vi "example_02_convert.vi"() -> ()   [LabVIEW 2015, in "lv-unit-conversion.lvlib"] (continued)
"d"=0.0, "underlying_def"="", "description"=""}, {"symbol"="GS", "name"="gigasiemens", "dimension"="I2T3/L2M", "is_si_unit"=TRUE, "category"="prefixed", "base_unit"="S", "conversion_reference"="DERIVED", "is_exact"=TRUE, "a"=0.0, "b"=1000000000.0, "c"=1.0, "d"=0.0, "underlying_def"="", "description"=""}, {"symbol"="kS", "name"="kilosiemens", "dimension"="I2T3/L2M", "is_si_unit"=TRUE, "category"="prefixed", "base_unit"="S", "conversion_reference"="DERIVED", "is_exact"=TRUE, "a"=0.0, "b"=1000.0, "c"=1.0, "d"=0.0, "underlying_def"="", "description"=""}, {"symbol"="mS", "name"="millisiemens", "dimension"="I2T3/L2M", "is_si_unit"=TRUE, "category"="prefixed", "base_unit"="S", "conversion_reference"="DERIVED", "is_exact"=TRUE, "a"=0.0, "b"=0.001, "c"=1.0, "d"=0.0, "underlying_def"="", "description"=""}, {"symbol"="MS", "name"="megasiemens", "dimension"="I2T3/L2M", "is_si_unit"=TRUE, "category"="prefixed", "base_unit"="S", "conversion_reference"="DERIVED", "is_exact"=TRUE, "a"=0.0, "b"=1000000.0, "c"=1.0, "d"=0.0, "underlying_def"="", "description"=""}, {"symbol"="nS", "name"="nanosiemens", "dimension"="I2T3/L2M", "is_si_unit"=TRUE, "category"="prefixed", "base_unit"="S", "conversion_reference"="DERIVED", "is_exact"=TRUE, "a"=0.0, "b"=1e-09, "c"=1.0, "d"=0.0, "underlying_def"="", "description"=""}, {"symbol"="pS", "name"="picosiemens", "dimension"="I2T3/L2M", "is_si_unit"=TRUE, "category"="prefixed", "base_unit"="S", "conversion_reference"="DERIVED", "is_exact"=TRUE, "a"=0.0, "b"=1e-12, "c"=1.0, "d"=0.0, "underlying_def"="", "description"=""}, {"symbol"="TS", "name"="terasiemens", "dimension"="I2T3/L2M", "is_si_unit"=TRUE, "category"="prefixed", "base_unit"="S", "conversion_reference"="DERIVED", "is_exact"=TRUE, "a"=0.0, "b"=1000000000000.0, "c"=1.0, "d"=0.0, "underlying_def"="", "description"=""}, {"symbol"="uS", "name"="microsiemens", "dimension"="I2T3/L2M", "is_si_unit"=TRUE, "category"="prefixed", "base_unit"="S", "conversion_reference"="DERIVED", "is_exact"=TRUE, "a"=0.0, "b"=1e-06, "c"=1.0, "d"=0.0, "underlying_def"="", "description"=""}, {"symbol"="S/m", "name"="siemens per metre", "dimension"="I2T3/L3M", "is_si_unit"=TRUE, "category"="derived", "base_unit"="", "conversion_reference"="", "is_exact"=FALSE, "a"=0.0, "b"=0.0, "c"=0.0, "d"=0.0, "underlying_def"="", "description"=""}, {"symbol"="kS/m", "name"="kilosiemens per metre", "dimension"="I2T3/L3M", "is_si_unit"=TRUE, "category"="derived", "base_unit"="S/m", "conversion_reference"="DERIVED", "is_exact"=TRUE, "a"=0.0, "b"=1000.0, "c"=1.0, "d"=0.0, "underlying_def"="", "description"=""}, {"symbol"="mS/cm", "name"="millisiemens per centimetre", "dimension"="I2T3/L3M", "is_si_unit"=TRUE, "category"="derived", "base_unit"="S/m", "conversion_reference"="DERIVED", "is_exact"=TRUE, "a"=0.0, "b"=0.1, "c"=1.0, "d"=0.0, "underlying_def"="", "description"=""}, {"symbol"="mS/m", "name"="millisiemens per metre", "dimension"="I2T3/L3M", "is_si_unit"=TRUE, "category"="derived", "base_unit"="S/m", "conversion_reference"="DERIVED", "is_exact"=TRUE, "a"=0.0, "b"=0.001, "c"=1.0, "d"=0.0, "underlying_def"="", "description"=""}, {"symbol"="F", "name"="farad", "dimension"="I2T4/L2M", "is_si_unit"=TRUE, "category"="atom-special", "base_unit"="", "conversion_reference"="", "is_exact"=FALSE, "a"=0.0, "b"=0.0, "c"=0.0, "d"=0.0, "underlying_def"="C/V", "description"="The capacitance of a capacitor between the plates of which there appears a difference of potential \n\t\t\t\tof 1 V when it is charged by a quantity of electricity equal to 1 C.\n\t\t\t"}, {"symbol"="cF", "name"="centifarad", "dimension"="I2T4/L2M", "is_si_unit"=TRUE, "category"="prefixed", "base_unit"="F", "conversion_reference"="DERIVED", "is_exact"=TRUE, "a"=0.0, "b"=0.01, "c"=1.0, "d"=0.0, "underlying_def"="", "description"=""}, {"symbol"="dF", "name"="decifarad", "dimension"="I2T4/L2M", "is_si_unit"=TRUE, "category"="prefixed", "base_unit"="F", "conversion_reference"="DERIVED", "is_exact"=TRUE, "a"=0.0, "b"=0.1, "c"=1.0, "d"=0.0, "underlying_def"="", "description"=""}, {"symbol"="EF", "name"="exafarad", "dimension"="I2T4/L2M", "is_si_unit"=TRUE, "category"="prefixed", "base_unit"="F", "conversion_reference"="DERIVED", "is_exact"=TRUE, "a"=0.0, "b"=1e+18, "c"=1.0, "d"=0.0, "underlying_def"="", "description"=""}, {"symbol"="fF", "name"="femtofarad", "dimension"="I2T4/L2M", "is_si_unit"=TRUE, "category"="prefixed", "base_unit"="F", "conversion_reference"="DERIVED", "is_exact"=TRUE, "a"=0.0, "b"=1e-15, "c"=1.0, "d"=0.0, "underlying_def"="", "description"=""}, {"symbol"="GF", "name"="gigafarad", "dimension"="I2T4/L2M", "is_si_unit"=TRUE, "category"="prefixed", "base_unit"="F", "conversion_reference"="DERIVED", "is_exact"=TRUE, "a"=0.0, "b"=1000000000.0, "c"=1.0, "d"=0.0, "underlying_def"="", "description"=""}, {"symbol"="kF", "name"="kilofarad", "dimension"="I2T4/L2M", "is_si_unit"=TRUE, "category"="prefixed", "base_unit"="F", "conversion_reference"="DERIVED", "is_exact"=TRUE, "a"=0.0, "b"=1000.0, "c"=1.0, "d"=0.0, "underlying_def"="", "description"=""}, {"symbol"="mF", "name"="millifarad", "dimension"="I2T4/L2M", "is_si_unit"=TRUE, "category"="prefixed", "base_unit"="F", "conversion_reference"="DERIVED", "is_exact"=TRUE, "a"=0.0, "b"=0.001, "c"=1.0, "d"=0.0, "underlying_def"="", "description"=""}, {"symbol"="MF", "name"="megafarad", "dimension"="I2T4/L2M", "is_si_unit"=TRUE, "category"="prefixed", "base_unit"="F", "conversion_reference"="DERIVED", "is_exact"=TRUE, "a"=0.0, "b"=1000000.0, "c"=1.0, "d"=0.0, "underlying_def"="", "description"=""}, {"symbol"="nF", "name"="nanofarad", "dimension"="I2T4/L2M", "is_si_unit"=TRUE, "category"="prefixed", "base_unit"="F", "conversion_reference"="DERIVED", "is_exact"=TRUE, "a"=0.0, "b"=1e-09, "c"=1.0, "d"=0.0, "underlying_def"="", "description"=""}, {"symbol"="pF", "name"="picofarad", "dimension"="I2T4/L2M", "is_si_unit"=TRUE, "category"="prefixed", "base_unit"="F", "conversion_reference"="DERIVED", "is_exact"=TRUE, "a"=0.0, "b"=1e-12, "c"=1.0, "d"=0.0, "underlying_def"="", "description"=""}, {"symbol"="TF", "name"="terafarad", "dimension"="I2T4/L2M", "is_si_unit"=TRUE, "category"="prefixed", "base_unit"="F", "conversion_reference"="DERIVED", "is_exact"=TRUE, "a"=0.0, "b"=1000000000000.0, "c"=1.0, "d"=0.0, "underlying_def"="", "description"=""}, {"symbol"="uF", "name"="microfarad", "dimension"="I2T4/L2M", "is_si_unit"=TRUE, "category"="prefixed", "base_unit"="F", "conversion_reference"="DERIVED", "is_exact"=TRUE, "a"=0.0, "b"=1e-06, "c"=1.0, "d"=0.0, "underlying_def"="", "description"=""}, {"symbol"="uF/m", "name"="microfarad per metre", "dimension"="I2T4/L3M", "is_si_unit"=TRUE, "category"="derived", "base_unit"="F/m", "conversion_reference"="DERIVED", "is_exact"=TRUE, "a"=0.0, "b"=1e-06, "c"=1.0, "d"=0.0, "underlying_def"="", "description"=""}, {"symbol"="F/m", "name"="farad per metre", "dimension"="I2T4/L3M", "is_si_unit"=TRUE, "category"="derived", "base_unit"="", "conversion_reference"="", "is_exact"=FALSE, "a"=0.0, "b"=0.0, "c"=0.0, "d"=0.0, "underlying_def"="", "description"=""}, {"symbol"="A.m2", "name"="ampere square metre", "dimension"="IL2", "is_si_unit"=TRUE, "category"="derived", "base_unit"="", "conversion_reference"="", "is_exact"=FALSE, "a"=0.0, "b"=0.0, "c"=0.0, "d"=0.0, "underlying_def"="", "description"=""}, {"symbol"="C.m", "name"="coulomb metre", "dimension"="ILT", "is_si_unit"=TRUE, "category"="derived", "base_unit"="", "conversion_reference"="", "is_exact"=FALSE, "a"=0.0, "b"=0.0, "c"=0.0, "d"=0.0, "underlying_def"="", "description"=""}, {"symbol"="C", "name"="coulomb", "dimension"="IT", "is_si_unit"=TRUE, "category"="atom-special", "base_unit"="", "conversion_reference"="", "is_exact"=FALSE, "a"=0.0, "b"=0.0, "c"=0.0, "d"=0.0, "underlying_def"="A.s", "description"="The time integral of electric current, equal to 1 A.s"}, {"symbol"="A.h", "name"="ampere hour", "dimension"="IT", "is_si_unit"=TRUE, "category"="derived", "base_unit"="C", "conversion_reference"="DERIVED", "is_exact"=TRUE, "a"=0.0, "b"=3600.0, "c"=1.0, "d"=0.0, "underlying_def"="", "description"=""}, {"symbol"="A.s", "name"="ampere second", "dimension"="IT", "is_si_unit"=TRUE, "category"="derived", "base_unit"="C", "conversion_reference"="DERIVED", "is_exact"=TRUE, "a"=0.0, "b"=1.0, "c"=1.0, "d"=0.0, "underlying_def"="", "description"=""}, {"symbol"="cC", "name"="centicoulomb", "dimension"="IT", "is_si_unit"=TRUE, "category"="prefixed", "base_unit"="C", "conversion_reference"="DERIVED", "is_exact"=TRUE, "a"=0.0, "b"=0.01, "c"=1.0, "d"=0.0, "underlying_def"="", "description"=""}, {"symbol"="dC", "name"="decicoulomb", "dimension"="IT", "is_si_unit"=TRUE, "category"="prefixed", "base_unit"="C", "conversion_reference"="DERIVED", "is_exact"=TRUE, "a"=0.0, "b"=0.1, "c"=1.0, "d"=0.0, "underlying_def"="", "description"=""}, {"symbol"="EC", "name"="exacoulomb", "dimension"="IT", "is_si_unit"=TRUE, "category"="prefixed", "base_unit"="C", "conversion_reference"="DERIVED", "is_exact"=TRUE, "a"=0.0, "b"=1e+18, "c"=1.0, "d"=0.0, "underlying_def"="", "description"=""}, {"symbol"="fC", "name"="femtocoulomb", "dimension"="IT", "is_si_unit"=TRUE, "category"="prefixed", "base_unit"="C", "conversion_reference"="DERIVED", "is_exact"=TRUE, "a"=0.0, "b"=1e-15, "c"=1.0, "d"=0.0, "underlying_def"="", "description"=""}, {"symbol"="GC", "name"="gigacoulomb", "dimension"="IT", "is_si_unit"=TRUE, "category"="prefixed", "base_unit"="C", "conversion_reference"="DERIVED", "is_exact"=TRUE, "a"=0.0, "b"=1000000000.0, "c"=1.0, "d"=0.0, "underlying_def"="", "description"=""}, {"symbol"="kC", "name"="kilocoulomb", "dimension"="IT", "is_si_unit"=TRUE, "category"="prefixed", "base_unit"="C", "conversion_reference"="DERIVED", "is_exact"=TRUE, "a"=0.0, "b"=1000.0, "c"=1.0, "d"=0.0, "underlying_def"="", "description"=""}, {"symbol"="mC", "name"="millicoulomb", "dimension"="IT", "is_si_unit"=TRUE, "category"="prefixed", "base_unit"="C", "conversion_reference"="DERIVED", "is_exact"=TRUE, "a"=0.0, "b"=0.001, "c"=1.0, "d"=0.0, "underlying_def"="", "description"=""}, {"symbol"="MC", "name"="megacoulomb", "dimension"="IT", "is_si_unit"=TRUE, "category"="prefixed", "base_unit"="C", "conversion_reference"="DERIVED", "is_exact"=TRUE, "a"=0.0, "b"=1000000.0, "c"=1.0, "d"=0.0, "underlying_def"="", "description"=""}, {"symbol"="nC", "name"="nanocoulomb", "dimension"="IT", "is_si_unit"=TRUE, "category"="prefixed", "base_unit"="C", "conversion_reference"="DERIVED", "is_exact"=TRUE, "a"=0.0, "b"=1e-09, "c"=1.0, "d"=0.0, "underlying_def"="", "description"=""}, {"symbol"="pC", "name"="picocoulomb", "dimension"="IT", "is_si_unit"=TRUE, "category"="prefixed", "base_unit"="C", "conversion_reference"="DERIVED", "is_exact"=TRUE, "a"=0.0, "b"=1e-12, "c"=1.0, "d"=0.0, "underlying_def"="", "description"=""}, {"symbol"="TC", "name"="teracoulomb", "dimension"="IT", "is_si_unit"=TRUE, "category"="prefixed", "base_unit"="C", "conversion_reference"="DERIVED", "is_exact"=TRUE, "a"=0.0, "b"=1000000000000.0, "c"=1.0, "d"=0.0, "underlying_def"="", "description"=""}, {"symbol"="uC", "name"="microcoulomb", "dimension"="IT", "is_si_unit"=TRUE, "category"="prefixed", "base_unit"="C", "conversion_reference"="DERIVED", "is_exact"=TRUE, "a"=0.0, "b"=1e-06, "c"=1.0, "d"=0.0, "underlying_def"="", "description"=""}, {"symbol"="C/cm2", "name"="coulomb per square centimetre", "dimension"="IT/L2", "is_si_unit"=TRUE, "category"="derived", "base_unit"="C/m2", "conversion_reference"="DERIVED", "is_exact"=TRUE, "a"=0.0, "b"=10000.0, "c"=1.0, "d"=0.0, "underlying_def"="", "description"=""}, {"symbol"="C/mm2", "name"="coulomb per square millimetre", "dimension"="IT/L2", "is_si_unit"=TRUE, "category"="derived", "base_unit"="C/m2", "conversion_reference"="DERIVED", "is_exact"=TRUE, "a"=0.0, "b"=1000000.0, "c"=1.0, "d"=0.0, "underlying_def"="", "description"=""}, {"symbol"="mC/m2", "name"="millicoulomb per square metre", "dimension"="IT/L2", "is_si_unit"=TRUE, "category"="derived", "base_unit"="C/m2", "conversion_reference"="DERIVED", "is_exact"=TRUE, "a"=0.0, "b"=0.001, "c"=1.0, "d"=0.0, "underlying_def"="", "description"=""}, {"symbol"="C/m2", "name"="coulomb per square metre", "dimension"="IT/L2", "is_si_unit"=TRUE, "category"="derived", "base_unit"="", "conversion_reference"="", "is_exact"=FALSE, "a"=0.0, "b"=0.0, "c"=0.0, "d"=0.0, "underlying_def"="", "description"=""}, {"symbol"="A.s/m3", "name"="ampere second per cubic metre", "dimension"="IT/L3", "is_si_unit"=TRUE, "category"="derived", "base_unit"="C/m3", "conversion_reference"="DERIVED", "is_exact"=TRUE, "a"=0.0, "b"=1.0, "c"=1.0, "d"=0.0, "underlying_def"="", "description"=""}, {"symbol"="C/cm3", "name"="coulomb per cubic centimetre", "dimension"="IT/L3", "is_si_unit"=TRUE, "category"="derived", "base_unit"="C/m3", "conversion_reference"="DERIVED", "is_exact"=TRUE, "a"=0.0, "b"=1000000.0, "c"=1.0, "d"=0.0, "underlying_def"="", "description"=""}, {"symbol"="C/mm3", "name"="coulomb per cubic millimetre", "dimension"="IT/L3", "is_si_unit"=TRUE, "category"="derived", "base_unit"="C/m3", "conversion_reference"="DERIVED", "is_exact"=TRUE, "a"=0.0, "b"=1000000000.0, "c"=1.0, "d"=0.0, "underlying_def"="", "description"=""}, {"symbol"="C/m3", "name"="coulomb per cubic metre", "dimension"="IT/L3", "is_si_unit"=TRUE, "category"="derived", "base_unit"="", "conversion_reference"="", "is_exact"=FALSE, "a"=0.0, "b"=0.0, "c"=0.0, "d"=0.0, "underlying_def"="", "description"=""}, {"symbol"="A.s/kg", "name"="ampere second per kilogram", "dimension"="IT/M", "is_si_unit"=TRUE, "category"="derived", "base_unit"="C/kg", "conversion_reference"="DERIVED", "is_exact"=TRUE, "a"=0.0, "b"=1.0, "c"=1.0, "d"=0.0, "underlying_def"="", "description"=""}, {"symbol"="C/g", "name"="coulomb per gram", "dimension"="IT/M", "is_si_unit"=TRUE, "category"="derived", "base_unit"="C/kg", "conversion_reference"="DERIVED", "is_exact"=TRUE, "a"=0.0, "b"=1000.0, "c"=1.0, "d"=0.0, "underlying_def"="", "description"=""}, {"symbol"="C/kg", "name"="coulomb per kilogram", "dimension"="IT/M", "is_si_unit"=TRUE, "category"="derived", "base_unit"="", "conversion_reference"="", "is_exact"=FALSE, "a"=0.0, "b"=0.0, "c"=0.0, "d"=0.0, "underlying_def"="", "description"=""}, {"symbol"="1/uV", "name"="per microvolt", "dimension"="IT3/L2M", "is_si_unit"=TRUE, "category"="derived", "base_unit"="1/V", "conversion_reference"="DERIVED", "is_exact"=TRUE, "a"=0.0, "b"=1000000.0, "c"=1.0, "d"=0.0, "underlying_def"="", "description"=""}, {"symbol"="1/V", "name"="per volt", "dimension"="IT3/L2M", "is_si_unit"=TRUE, "category"="derived", "base_unit"="", "conversion_reference"="", "is_exact"=FALSE, "a"=0.0, "b"=0.0, "c"=0.0, "d"=0.0, "underlying_def"="", "description"=""}, {"symbol"="cd", "name"="candela", "dimension"="J", "is_si_unit"=TRUE, "category"="atom-base", "base_unit"="", "conversion_reference"="", "is_exact"=FALSE, "a"=0.0, "b"=0.0, "c"=0.0, "d"=0.0, "underlying_def"="", "description"="The candela is the luminous intensity, in a given direction, of a source that emits monochromatic \n\t\t\t\tradiation of frequency 540 X 10**12 hertz and that has a radian intensity in that direction of 1/683 \n\t\t\t\twatt per steradian.\n\t\t\t"}, {"symbol"="kcd", "name"="kilocandela", "dimension"="J", "is_si_unit"=TRUE, "category"="prefixed", "base_unit"="cd", "conversion_reference"="DERIVED", "is_exact"=TRUE, "a"=0.0, "b"=1000.0, "c"=1.0, "d"=0.0, "underlying_def"="", "description"=""}, {"symbol"="cd/m2", "name"="candela per square metre", "dimension"="J/L2", "is_si_unit"=TRUE, "category"="derived", "base_unit"="", "conversion_reference"="", "is_exact"=FALSE, "a"=0.0, "b"=0.0, "c"=0.0, "d"=0.0, "underlying_def"="", "description"=""}, {"symbol"="lm", "name"="lumen", "dimension"="JS", "is_si_unit"=TRUE, "category"="atom-special", "base_unit"="", "conversion_reference"="", "is_exact"=FALSE, "a"=0.0, "b"=0.0, "c"=0.0, "d"=0.0, "underlying_def"="cd.sr", "description"="The luminous flux emitted in a solid angle of 1 sr by a point source having a uniform intensity of 1 cd.\n\t\t\t"}, {"symbol"="lx", "name"="lux", "dimension"="JS/L2", "is_si_unit"=TRUE, "category"="atom-special", "base_unit"="", "conversion_reference"="", "is_exact"=FALSE, "a"=0.0, "b"=0.0, "c"=0.0, "d"=0.0, "underlying_def"="lm/m2", "description"="The illuminance produced by a luminous flux of 1 lm uniformly distributed over a surface of 1 m2."}, {"symbol"="footcandle", "name"="footcandle", "dimension"="JS/L2", "is_si_unit"=TRUE, "category"="atom", "base_unit"="lx", "conversion_reference"="DEFINITION", "is_exact"=TRUE, "a"=0.0, "b"=1.0, "c"=0.09290304, "d"=0.0, "underlying_def"="lm/ft2", "description"="A unit of illuminance on a surface that is everywhere one foot from a uniform point source of light \n\t\t\t\tof one candle and equal to one lumen per square foot (from www.merriam-webster.com). \n\t\t\t\tTo convert to Lux, convert the square foot component to square meter (i.e., 1/( 0.3048)**2).\n\t\t\t"}, {"symbol"="lm/m2", "name"="lumen per square metre", "dimension"="JS/L2", "is_si_unit"=TRUE, "category"="derived", "base_unit"="lx", "conversion_reference"="DERIVED", "is_exact"=TRUE, "a"=0.0, "b"=1.0, "c"=1.0, "d"=0.0, "underlying_def"="", "description"=""}, {"symbol"="klx", "name"="kilolux", "dimension"="JS/L2", "is_si_unit"=TRUE, "category"="prefixed", "base_unit"="lx", "conversion_reference"="DERIVED", "is_exact"=TRUE, "a"=0.0, "b"=1000.0, "c"=1.0, "d"=0.0, "underlying_def"="", "description"=""}, {"symbol"="lm.s", "name"="lumen second", "dimension"="JST", "is_si_unit"=TRUE, "category"="derived", "base_unit"="", "conversion_reference"="", "is_exact"=FALSE, "a"=0.0, "b"=0.0, "c"=0.0, "d"=0.0, "underlying_def"="", "description"="Also known as a talbot."}, {"symbol"="lx.s", "name"="lux second", "dimension"="JST/L2", "is_si_unit"=TRUE, "category"="derived", "base_unit"="", "conversion_reference"="", "is_exact"=FALSE, "a"=0.0, "b"=0.0, "c"=0.0, "d"=0.0, "underlying_def"="", "description"=""}, {"symbol"="footcandle.s", "name"="footcandle second", "dimension"="JST/L2", "is_si_unit"=TRUE, "category"="derived", "base_unit"="lx.s", "conversion_reference"="DERIVED", "is_exact"=TRUE, "a"=0.0, "b"=1.0, "c"=0.09290304, "d"=0.0, "underlying_def"="", "description"=""}, {"symbol"="lm/W", "name"="lumen per watt", "dimension"="JST3/L2M", "is_si_unit"=TRUE, "category"="derived", "base_unit"="", "conversion_reference"="", "is_exact"=FALSE, "a"=0.0, "b"=0.0, "c"=0.0, "d"=0.0, "underlying_def"="", "description"=""}, {"symbol"="K", "name"="degree kelvin", "dimension"="K", "is_si_unit"=TRUE, "category"="atom-base", "base_unit"="", "conversion_reference"="", "is_exact"=FALSE, "a"=0.0, "b"=0.0, "c"=0.0, "d"=0.0, "underlying_def"="", "description"="The kelvin, unit of thermodynamic temperature, is the fraction 1/273.16 of the thermodynamic \n\t\t\t\ttemperature of the triple point of water.\n\t\t\t"}, {"symbol"="degC", "name"="degree Celsius", "dimension"="K", "is_si_unit"=TRUE, "category"="atom-special", "base_unit"="K", "conversion_reference"="NIST-SI", "is_exact"=TRUE, "a"=273.15, "b"=1.0, "c"=1.0, "d"=0.0, "underlying_def"="", "description"="Kelvin minus 273.15"}, {"symbol"="degF", "name"="degree Fahrenheit", "dimension"="K", "is_si_unit"=TRUE, "category"="atom", "base_unit"="K", "conversion_reference"="NIST-SI", "is_exact"=TRUE, "a"=2298.35, "b"=5.0, "c"=9.0, "d"=0.0, "underlying_def"="", "description"="Kelvin=(Fahrenheit + 459.67)(5/9)"}, {"symbol"="degR", "name"="degree Rankine", "dimension"="K", "is_si_unit"=TRUE, "category"="atom", "base_unit"="K", "conversion_reference"="NIST-SI", "is_exact"=TRUE, "a"=0.0, "b"=5.0, "c"=9.0, "d"=0.0, "underlying_def"="", "description"="Kelvin=(Rankin)(5/9)"}, {"symbol"="m", "name"="metre", "dimension"="L", "is_si_unit"=TRUE, "category"="atom-base", "base_unit"="", "conversion_reference"="", "is_exact"=FALSE, "a"=0.0, "b"=0.0, "c"=0.0, "d"=0.0, "underlying_def"="", "description"="The metre is the length equal to 1 650 763.73 wavelengths in vacuum of the radiation corresponding \n\t\t\t\tto the transition between the levels 2p10 and 5d5 of the krypton-86 atom. \n\t\t\t\tIn the US, this is called a meter.\n\t\t\t"}, {"symbol"="angstrom", "name"="angstrom", "dimension"="L", "is_si_unit"=TRUE, "category"="atom-allowed", "base_unit"="m", "conversion_reference"="NIST-SI", "is_exact"=TRUE, "a"=0.0, "b"=1e-10, "c"=1.0, "d"=0.0, "underlying_def"="0.1 nm", "description"="The angstrom is widely used by x-ray crystallographers and structural chemists because all chemical \n\t\t\t\tbonds lie in the range 1 to 3 angstroms.\n\t\t\t"}, {"symbol"="chain", "name"="chain", "dimension"="L", "is_si_unit"=TRUE, "category"="atom", "base_unit"="m", "conversion_reference"="EPSG", "is_exact"=TRUE, "a"=0.0, "b"=20.1168, "c"=1.0, "d"=0.0, "underlying_def"="66 ft", "description"="international chain equal to 22 international yards or 66 international feet. From EPSG."}, {"symbol"="chain[BnA]", "name"="British chain [Benoit 1895 A]", "dimension"="L", "is_si_unit"=TRUE, "category"="atom", "base_unit"="m", "conversion_reference"="EPSG", "is_exact"=TRUE, "a"=0.0, "b"=20.1167824, "c"=1.0, "d"=0.0, "underlying_def"="66 ft[BnA]", "description"="66 British foot [Benoit 1895 A]"}, {"symbol"="chain[BnB]", "name"="British chain [Benoit 1895 B]", "dimension"="L", "is_si_unit"=TRUE, "category"="atom", "base_unit"="m", "conversion_reference"="EPSG", "is_exact"=TRUE, "a"=0.0, "b"=792.0, "c"=39.370113, "d"=0.0, "underlying_def"="66 ft[BnB]", "description"="66 British foot [Benoit 1895 B]"}, {"symbol"="chain[Cla]", "name"="Clarke chain", "dimension"="L", "is_si_unit"=TRUE, "category"="atom", "base_unit"="m", "conversion_reference"="EPSG", "is_exact"=TRUE, "a"=0.0, "b"=20.1166195164, "c"=1.0, "d"=0.0, "underlying_def"="66 ft[Cla]", "description"="66 Clarke foot"}, {"symbol"="chain[Ind37]", "name"="Indian Chain [1937]", "dimension"="L", "is_si_unit"=TRUE, "category"="atom", "base_unit"="m", "conversion_reference"="DEFINITION", "is_exact"=TRUE, "a"=0.0, "b"=20.11669506, "c"=1.0, "d"=0.0, "underlying_def"="66 ft[Ind37]", "description"="66 Indian foot [1937]"}, {"symbol"="chain[Se]", "name"="British chain [Sears 1922]", "dimension"="L", "is_si_unit"=TRUE, "category"="atom", "base_unit"="m", "conversion_reference"="EPSG", "is_exact"=TRUE, "a"=0.0, "b"=792.0, "c"=39.370147, "d"=0.0, "underlying_def"="66 ft[Se]", "description"="66 British foot [Sears 1922]"}, {"symbol"="chain[SeT]", "name"="British chain [Sears 1922 truncated]", "dimension"="L", "is_si_unit"=TRUE, "category"="atom", "base_unit"="m", "conversion_reference"="EPSG", "is_exact"=TRUE, "a"=0.0, "b"=20.116756, "c"=1.0, "d"=0.0, "underlying_def"="66 ft[SeT]", "description"="66 British foot [Sears 1922 truncated]"}, {"symbol"="chain[US]", "name"="US survey chain", "dimension"="L", "is_si_unit"=TRUE, "category"="atom", "base_unit"="m", "conversion_reference"="EPSG", "is_exact"=TRUE, "a"=0.0, "b"=792.0, "c"=39.37, "d"=0.0, "underlying_def"="66 ft[US]", "description"="66 US survey feet (exactly). Also called Gunter's chain. From NIST-44."}, {"symbol"="fathom", "name"="international fathom", "dimension"="L", "is_si_unit"=TRUE, "category"="atom", "base_unit"="m", "conversion_reference"="EPSG", "is_exact"=TRUE, "a"=0.0, "b"=1.8288, "c"=1.0, "d"=0.0, "underlying_def"="6 ft", "description"="6 international foot."}, {"symbol"="ft", "name"="foot", "dimension"="L", "is_si_unit"=TRUE, "category"="atom", "base_unit"="m", "conversion_reference"="NIST-SI", "is_exact"=TRUE, "a"=0.0, "b"=0.3048, "c"=1.0, "d"=0.0, "underlying_def"="1/3 yd", "description"="International foot"}, {"symbol"="ft[BnA]", "name"="British foot [Benoit 1895 A]", "dimension"="L", "is_si_unit"=TRUE, "category"="atom", "base_unit"="m", "conversion_reference"="EPSG", "is_exact"=TRUE, "a"=0.0, "b"=0.9143992, "c"=3.0, "d"=0.0, "underlying_def"="", "description"="Uses Benoit's 1895 British yard-metre ratio as given by Clark as 0.9143992 metre.s per yard. \n\t\t\t\tUsed for deriving metric size of ellipsoid in Palestine.\n\t\t\t"}, {"symbol"="ft[BnB]", "name"="British foot [Benoit 1895 B]", "dimension"="L", "is_si_unit"=TRUE, "category"="atom", "base_unit"="m", "conversion_reference"="EPSG", "is_exact"=TRUE, "a"=0.0, "b"=12.0, "c"=39.370113, "d"=0.0, "underlying_def"="", "description"="Uses Benoit's 1895 British yard-metre ratio as given by Bomford as 39.370113 inches per metre. \n\t\t\t\tUsed in West Malaysian mapping.\n\t\t\t"}, {"symbol"="ft[Br36]", "name"="British foot [1936]", "dimension"="L", "is_si_unit"=TRUE, "category"="atom", "base_unit"="m", "conversion_reference"="EPSG", "is_exact"=TRUE, "a"=0.0, "b"=0.3048007491, "c"=1.0, "d"=0.0, "underlying_def"="", "description"="For the 1936 retriangulation OSGB defines the relationship of 10 feet of 1796 to the International \n\t\t\t\tmetre through the logarithmic relationship (10^0.48401603 exactly). \n\t\t\t\t1 ft = 0.3048007491...m. \n\t\t\t\tAlso used for metric conversions in Ireland.\n\t\t\t"}, {"symbol"="ft[Br65]", "name"="British foot [1865]", "dimension"="L", "is_si_unit"=TRUE, "category"="atom", "base_unit"="m", "conversion_reference"="EPSG", "is_exact"=TRUE, "a"=0.0, "b"=0.9144025, "c"=3.0, "d"=0.0, "underlying_def"="", "description"="Uses Clark's estimate of 1853-1865 British foot-metre ratio of 0.9144025 metres per yard. \n\t\t\t\tUsed in 1962 and 1975 estimates of Indian foot.\n\t\t\t"}, {"symbol"="ft[Cla]", "name"="Clarke foot", "dimension"="L", "is_si_unit"=TRUE, "category"="atom", "base_unit"="m", "conversion_reference"="EPSG", "is_exact"=TRUE, "a"=0.0, "b"=0.3047972654, "c"=1.0, "d"=0.0, "underlying_def"="", "description"="Assumes Clarke's 1865 ratio of 1 British foot = 0.3047972654 French legal metres applies to the \n\t\t\t\tinternational metre.\n\t\t\t"}, {"symbol"="ft[GC]", "name"="Gold Coast foot", "dimension"="L", "is_si_unit"=TRUE, "category"="atom", "base_unit"="m", "conversion_reference"="EPSG", "is_exact"=TRUE, "a"=0.0, "b"=6378300.0, "c"=20926201.0, "d"=0.0, "underlying_def"="", "description"="Used in Ghana and some adjacent parts of British west Africa prior to metrication, except for the \n\t\t\t\tmetrication of projection defining parameters when British foot (Sears 1922) used.\n\t\t\t"}, {"symbol"="ft[Ind]", "name"="indian foot", "dimension"="L", "is_si_unit"=TRUE, "category"="atom", "base_unit"="m", "conversion_reference"="EPSG", "is_exact"=TRUE, "a"=0.0, "b"=12.0, "c"=39.370142, "d"=0.0, "underlying_def"="", "description"="Indian Foot = 0.99999566 British feet (A.R.Clarke 1865). \n\t\t\t\tBritish yard (= 3 British feet) taken to be J.S.Clark's 1865 value of 0.9144025 metres.\n\t\t\t"}, {"symbol"="ft[Ind37]", "name"="indian foot [1937]", "dimension"="L", "is_si_unit"=TRUE, "category"="atom", "base_unit"="m", "conversion_reference"="EPSG", "is_exact"=TRUE, "a"=0.0, "b"=0.30479841, "c"=1.0, "d"=0.0, "underlying_def"="", "description"="Indian Foot = 0.99999566 British feet (A.R.Clarke 1865). \n\t\t\t\tBritish foot taken to be 1895 Benoit value of 12/39.370113m. \n\t\t\t\tRounded to 8 decimal places as 0.30479841. \n\t\t\t\tUsed from Bangladesh to Vietnam. \n\t\t\t\tPreviously used in India and Pakistan but superseded.\n\t\t\t"}, {"symbol"="ft[Ind62]", "name"="indian foot ]1962]", "dimension"="L", "is_si_unit"=TRUE, "category"="atom", "base_unit"="m", "conversion_reference"="EPSG", "is_exact"=TRUE, "a"=0.0, "b"=0.3047996, "c"=1.0, "d"=0.0, "underlying_def"="", "description"="Indian Foot = 0.99999566 British feet (A.R.Clarke 1865). \n\t\t\t\tBritish yard (3 feet) taken to be J.S. \n\t\t\t\tClark's 1865 value of 0.9144025m. \n\t\t\t\tRounded to 7 significant figures with a small error as 1 Ind ft=0.3047996m. \n\t\t\t\tUsed in Pakistan since metrication.\n\t\t\t"}, {"symbol"="ft[Ind75]", "name"="indian foot [1975]", "dimension"="L", "is_si_unit"=TRUE, "category"="atom", "base_unit"="m", "conversion_reference"="EPSG", "is_exact"=TRUE, "a"=0.0, "b"=0.3047995, "c"=1.0, "d"=0.0, "underlying_def"="", "description"="Indian Foot = 0.99999566 British feet (A.R.Clarke 1865). \n\t\t\t\tBritish yard (3 feet) taken to be J.S. \n\t\t\t\tClark's 1865 value of 0.9144025m. \n\t\t\t\tRounded to 7 significant figures as 1 Ind ft=0.3047995m. \n\t\t\t\tUsed in India since metrication.\n\t\t\t"}, {"symbol"="ft[Se]", "name"="British foot [Sears 1922]", "dimension"="L", "is_si_unit"=TRUE, "category"="atom", "base_unit"="m", "conversion_reference"="EPSG", "is_exact"=TRUE, "a"=0.0, "b"=12.0, "c"=39.370147, "d"=0.0, "underlying_def"="", "description"="Uses Sear's 1922 British yard-metre ratio as given by Bomford as 39.370147 inches per metre. \n\t\t\t\tUsed in East Malaysian and older New Zealand mapping.\n\t\t\t"}, {"symbol"="ft[SeT]", "name"="British foot [Sears 1922 truncated]", "dimension"="L", "is_si_unit"=TRUE, "category"="atom", "base_unit"="m", "conversion_reference"="EPSG", "is_exact"=TRUE, "a"=0.0, "b"=0.914398, "c"=3.0, "d"=0.0, "underlying_def"="", "description"="Uses Sear's 1922 British yard-metre ratio (UoM code 9040) truncated to 6 significant figures; this \n\t\t\t\ttruncated ratio (0.914398, UoM code 9099) then converted to other imperial units. \n\t\t\t\t3 ftSe(T) = 1 ydSe(T).\n\t\t\t"}, {"symbol"="ft[US]", "name"="US survey foot", "dimension"="L", "is_si_unit"=TRUE, "category"="atom", "base_unit"="m", "conversion_reference"="NIST-SI", "is_exact"=TRUE, "a"=0.0, "b"=1200.0, "c"=3937.0, "d"=0.0, "underlying_def"="1200/3937 m", "description"="Used in USA."}, {"symbol"="fur[US]", "name"="furlong US survey", "dimension"="L", "is_si_unit"=TRUE, "category"="atom", "base_unit"="m", "conversion_reference"="NIST-44", "is_exact"=TRUE, "a"=0.0, "b"=792000.0, "c"=3937.0, "d"=0.0, "underlying_def"="660 ft[US]", "description"="660 US survey foot (exactly)."}, {"symbol"="in", "name"="inch", "dimension"="L", "is_si_unit"=TRUE, "category"="atom", "base_unit"="m", "conversion_reference"="NIST-SI", "is_exact"=TRUE, "a"=0.0, "b"=0.0254, "c"=1.0, "d"=0.0, "underlying_def"="2.54 cm", "description"="international inch"}, {"symbol"="in[US]", "name"="US survey inch", "dimension"="L", "is_si_unit"=TRUE, "category"="atom", "base_unit"="m", "conversion_reference"="NIST-SI", "is_exact"=TRUE, "a"=0.0, "b"=100.0, "c"=3937.0, "d"=0.0, "underlying_def"="1/12 ft[US]", "description"="1/12 of US survey foot."}, {"symbol"="link", "name"="link", "dimension"="L", "is_si_unit"=TRUE, "category"="atom", "base_unit"="m", "conversion_reference"="EPSG", "is_exact"=TRUE, "a"=0.0, "b"=20.1168, "c"=100.0, "d"=0.0, "underlying_def"="1/100 chain", "description"="66/100 international foot. 1/100 international chain."}, {"symbol"="link[BnA]", "name"="British link [Benoit 1895 A]", "dimension"="L", "is_si_unit"=TRUE, "category"="atom", "base_unit"="m", "conversion_reference"="EPSG", "is_exact"=TRUE, "a"=0.0, "b"=0.201167824, "c"=1.0, "d"=0.0, "underlying_def"="1/100 chain[BnA]", "description"="66/100 British foot [Benoit 1895 A]"}, {"symbol"="link[BnB]", "name"="British link [Benoit 1895 B]", "dimension"="L", "is_si_unit"=TRUE, "category"="atom", "base_unit"="m", "conversion_reference"="EPSG", "is_exact"=TRUE, "a"=0.0, "b"=7.92, "c"=39.370113, "d"=0.0, "underlying_def"="1/100 chain[BnB]", "description"="66/100 British foot [Benoit 1895 B]"}, {"symbol"="link[Cla]", "name"="Clarke link", "dimension"="L", "is_si_unit"=TRUE, "category"="atom", "base_unit"="m", "conversion_reference"="EPSG", "is_exact"=TRUE, "a"=0.0, "b"=0.201166195164, "c"=1.0, "d"=0.0, "underlying_def"="1/100 chain[Cla]", "description"="66/100 Clarke foot"}, {"symbol"="link[Se]", "name"="British link [Sears 1922]", "dimension"="L", "is_si_unit"=TRUE, "category"="atom", "base_unit"="m", "conversion_reference"="EPSG", "is_exact"=TRUE, "a"=0.0, "b"=7.92, "c"=39.370147, "d"=0.0, "underlying_def"="1/100 chain[Se]", "description"="66/100 British foot [Sears 1922]"}, {"symbol"="link[SeT]", "name"="British link [Sears 1922 truncated]", "dimension"="L", "is_si_unit"=TRUE, "category"="atom", "base_unit"="m", "conversion_reference"="EPSG", "is_exact"=TRUE, "a"=0.0, "b"=0.20116756, "c"=1.0, "d"=0.0, "underlying_def"="1/100 chain[SeT]", "description"="66/100 British foot (Sears 1922 truncated)"}, {"symbol"="link[US]", "name"="US survey link", "dimension"="L", "is_si_unit"=TRUE, "category"="atom", "base_unit"="m", "conversion_reference"="NIST-44", "is_exact"=TRUE, "a"=0.0, "b"=7.92, "c"=39.37, "d"=0.0, "underlying_def"="1/100 chain[US]", "description"="US survey link. Equal to 0.66 US survey foot (exactly)."}, {"symbol"="m[Ger]", "name"="German legal metre", "dimension"="L", "is_si_unit"=TRUE, "category"="atom", "base_unit"="m", "conversion_reference"="EPSG", "is_exact"=TRUE, "a"=0.0, "b"=1.0000135965, "c"=1.0, "d"=0.0, "underlying_def"="", "description"="Used in Namibia."}, {"symbol"="mi", "name"="mile", "dimension"="L", "is_si_unit"=TRUE, "category"="atom", "base_unit"="m", "conversion_reference"="NIST-44", "is_exact"=TRUE, "a"=0.0, "b"=1609.344, "c"=1.0, "d"=0.0, "underlying_def"="5280 ft", "description"="International mile."}, {"symbol"="mi[naut]", "name"="international nautical mile", "dimension"="L", "is_si_unit"=TRUE, "category"="atom-allowed", "base_unit"="m", "conversion_reference"="NIST-SI", "is_exact"=TRUE, "a"=0.0, "b"=1852.0, "c"=1.0, "d"=0.0, "underlying_def"="1852 m", "description"="The nautical mile is a special unit employed for marine and aerial navigation to express distance. \n\t\t\t\tThe unit was originally chosen, and continues to be used, because one nautical mile on the surface \n\t\t\t\tof the Earth subtends approximately one minute of angle at the centre of the Earth, which is \n\t\t\t\tconvenient when latitude and longitude are measured in degrees and minutes of angle.\n\t\t\t"}, {"symbol"="mi[nautUK]", "name"="United Kingdom nautical mile", "dimension"="L", "is_si_unit"=TRUE, "category"="atom", "base_unit"="m", "conversion_reference"="UK-1995", "is_exact"=TRUE, "a"=0.0, "b"=1853.0, "c"=1.0, "d"=0.0, "underlying_def"="1853 m", "description"="The Imperial (UK) nautical mile, also known as the Admiralty mile, was defined in terms of the knot, \n\t\t\t\tsuch that one nautical mile was exactly 6,080 international feet (1,853.184 m):[6] it was abandoned \n\t\t\t\tin 1970[6] and, for legal purposes, old references to the obsolete unit are now converted to 1,853 \n\t\t\t\tmetres exactly.\n\t\t\t"}, {"symbol"="mi[US]", "name"="US survey mile", "dimension"="L", "is_si_unit"=TRUE, "category"="atom", "base_unit"="m", "conversion_reference"="NIST-44", "is_exact"=TRUE, "a"=0.0, "b"=6336000.0, "c"=3937.0, "d"=0.0, "underlying_def"="5280 ft[US]", "description"="United States survey mile is 5280 feet survey (exactly). From NIST-55."}, {"symbol"="mil", "name"="mil", "dimension"="L", "is_si_unit"=TRUE, "category"="atom", "base_unit"="m", "conversion_reference"="NIST-44", "is_exact"=TRUE, "a"=0.0, "b"=2.54e-05, "c"=1.0, "d"=0.0, "underlying_def"="1/1000 in", "description"="One thousandth of an inch."}, {"symbol"="rod[US]", "name"="rod US Survey", "dimension"="L", "is_si_unit"=TRUE, "category"="atom", "base_unit"="m", "conversion_reference"="NIST-44", "is_exact"=TRUE, "a"=0.0, "b"=19800.0, "c"=3937.0, "d"=0.0, "underlying_def"="16.5 ft[US]", "description"="16.5 US survey feet (exactly)"}, {"symbol"="yd", "name"="yard", "dimension"="L", "is_si_unit"=TRUE, "category"="atom", "base_unit"="m", "conversion_reference"="NIST-44", "is_exact"=TRUE, "a"=0.0, "b"=0.9144, "c"=1.0, "d"=0.0, "underlying_def"="3 ft", "description"="International yard."}, {"symbol"="yd[BnA]", "name"="British yard [Benoit 1895 A]", "dimension"="L", "is_si_unit"=TRUE, "category"="atom", "base_unit"="m", "conversion_reference"="EPSG", "is_exact"=TRUE, "a"=0.0, "b"=0.9143992, "c"=1.0, "d"=0.0, "underlying_def"="3 ft[BnA]", "description"="3 British foot [Benoit 1895 A]"}, {"symbol"="yd[BnB]", "name"="British yard [Benoit 1895 B]", "dimension"="L", "is_si_unit"=TRUE, "category"="atom", "base_unit"="m", "conversion_reference"="EPSG", "is_exact"=TRUE, "a"=0.0, "b"=36.0, "c"=39.370113, "d"=0.0, "underlying_def"="3 ft[BnB]", "description"="3 British foot [Benoit 1895 B]"}, {"symbol"="yd[Cla]", "name"="Clarke yard", "dimension"="L", "is_si_unit"=TRUE, "category"="atom", "base_unit"="m", "conversion_reference"="EPSG", "is_exact"=TRUE, "a"=0.0, "b"=0.9143917962, "c"=1.0, "d"=0.0, "underlying_def"="3 ft[Cla]", "description"="3 Clark foot."}, {"symbol"="yd[Ind]", "name"="Indian yard", "dimension"="L", "is_si_unit"=TRUE, "category"="atom", "base_unit"="m", "conversion_reference"="EPSG", "is_exact"=TRUE, "a"=0.0, "b"=36.0, "c"=39.370142, "d"=0.0, "underlying_def"="3 ft[Ind]", "description"="3 Indian foot"}, {"symbol"="yd[Ind37]", "name"="Indian yard [1937]", "dimension"="L", "is_si_unit"=TRUE, "category"="atom", "base_unit"="m", "conversion_reference"="EPSG", "is_exact"=TRUE, "a"=0.0, "b"=0.91439523, "c"=1.0, "d"=0.0, "underlying_def"="3 ft[Ind37]", "description"="3 Indian foot [1937]"}, {"symbol"="yd[Ind62]", "name"="Indian yard [1962]", "dimension"="L", "is_si_unit"=TRUE, "category"="atom", "base_unit"="m", "conversion_reference"="EPSG", "is_exact"=TRUE, "a"=0.0, "b"=0.9143988, "c"=1.0, "d"=0.0, "underlying_def"="3 ft[Ind62]", "description"="3 Indian foot [1962]"}, {"symbol"="yd[Ind75]", "name"="Indian yard [1975]", "dimension"="L", "is_si_unit"=TRUE, "category"="atom", "base_unit"="m", "conversion_reference"="EPSG", "is_exact"=TRUE, "a"=0.0, "b"=0.9143985, "c"=1.0, "d"=0.0, "underlying_def"="3 ft[Ind75]", "description"="3 Indian foot [1975]"}, {"symbol"="yd[Se]", "name"="British yard [Sears 1922]", "dimension"="L", "is_si_unit"=TRUE, "category"="atom", "base_unit"="m", "conversion_reference"="EPSG", "is_exact"=TRUE, "a"=0.0, "b"=36.0, "c"=39.370147, "d"=0.0, "underlying_def"="3 ft[Se]", "description"="3 British foot [Sears 1922]"}, {"symbol"="yd[SeT]", "name"="British yard [Sears 1922 truncated]", "dimension"="L", "is_si_unit"=TRUE, "category"="atom", "base_unit"="m", "conversion_reference"="EPSG", "is_exact"=TRUE, "a"=0.0, "b"=0.914398, "c"=1.0, "d"=0.0, "underlying_def"="3 ft[SeT]", "description"="3 British foot [Sears 1922 truncated]"}, {"symbol"="yd[US]", "name"="US survey yard", "dimension"="L", "is_si_unit"=TRUE, "category"="atom", "base_unit"="m", "conversion_reference"="NIST-SI", "is_exact"=TRUE, "a"=0.0, "b"=3600.0, "c"=3937.0, "d"=0.0, "underlying_def"="3 ft[US]", "description"="3 US survey foot."}, {"symbol"="m3/m2", "name"="cubic metre per square metre", "dimension"="L", "is_si_unit"=TRUE, "category"="derived", "base_unit"="", "conversion_reference"="", "is_exact"=FALSE, "a"=0.0, "b"=0.0, "c"=0.0, "d"=0.0, "underlying_def"="m", "description"=""}, {"symbol"="0.1 ft", "name"="tenth of foot", "dimension"="L", "is_si_unit"=TRUE, "category"="derived", "base_unit"="m", "conversion_reference"="DERIVED", "is_exact"=TRUE, "a"=0.0, "b"=0.03048, "c"=1.0, "d"=0.0, "underlying_def"="", "description"=""}, {"symbol"="0.1 ft[US]", "name"="tenth of US survey foot", "dimension"="L", "is_si_unit"=TRUE, "category"="derived", "base_unit"="m", "conversion_reference"="DERIVED", "is_exact"=TRUE, "a"=0.0, "b"=1200.0, "c"=39370.0, "d"=0.0, "underlying_def"="", "description"=""}, {"symbol"="0.1 in", "name"="tenth of inch", "dimension"="L", "is_si_unit"=TRUE, "category"="derived", "base_unit"="m", "conversion_reference"="DERIVED", "is_exact"=TRUE, "a"=0.0, "b"=0.00254, "c"=1.0, "d"=0.0, "underlying_def"="", "description"=""}, {"symbol"="0.1 yd", "name"="tenth of yard", "dimension"="L", "is_si_unit"=TRUE, "category"="derived", "base_unit"="m", "conversion_reference"="DERIVED", "is_exact"=TRUE, "a"=0.0, "b"=0.09144, "c"=1.0, "d"=0.0, "underlying_def"="", "description"=""}, {"symbol"="1/16 in", "name"="sixteenth of inch", "dimension"="L", "is_si_unit"=TRUE, "category"="derived", "base_unit"="m", "conversion_reference"="DERIVED", "is_exact"=TRUE, "a"=0.0, "b"=0.0254, "c"=16.0, "d"=0.0, "underlying_def"="", "description"=""}, {"symbol"="1/2 ft", "name"="half of Foot", "dimension"="L", "is_si_unit"=TRUE, "category"="derived", "base_unit"="m", "conversion_reference"="DERIVED", "is_exact"=TRUE, "a"=0.0, "b"=0.3048, "c"=2.0, "d"=0.0, "underlying_def"="", "description"=""}, {"symbol"="1/32 
